vi "Analog Input Voltages.vi"(8 "error in (no error)":errorcluster, 10 "Analog Input Voltages":waveform(dbl)[](array[waveform]), 11 "BPG in":refnum<class "BPG.lvclass">) -> (0 "error out":errorcluster, 3 "BPG out":refnum<class "BPG.lvclass">)   [LabVIEW 2021, in "BPG.lvclass"]
uses:
  BPG.lvclass
  C:/Program Files/National Instruments/LabVIEW 2021/vi.lib/ActorFramework/Actor/Actor.lvclass
  <vilib>/NathanCo/Color Compare/Utilities/Colors.ctl
  BPG.lvclass/BPG.ctl
  <vilib>/ActorFramework/Actor/Actor.lvclass/Actor.ctl
  Pressure Gauges/Pressure Gauges Messages/Received Pressure Msg/Received Pressure Msg.lvclass/Received Pressure Msg.ctl
  <vilib>/ActorFramework/Message Enqueuer/Message Enqueuer.lvclass/Message Enqueuer.ctl
  <vilib>/ActorFramework/Message Enqueuer/Enqueue.vi
  Pressure Gauges/Pressure Gauges Messages/Received Pressure Msg/Received Pressure Msg.lvclass
  C:/Program Files/National Instruments/LabVIEW 2021/vi.lib/ActorFramework/Message/Message.lvclass
  <vilib>/ActorFramework/Message Priority Queue/Priority Enqueue.vi
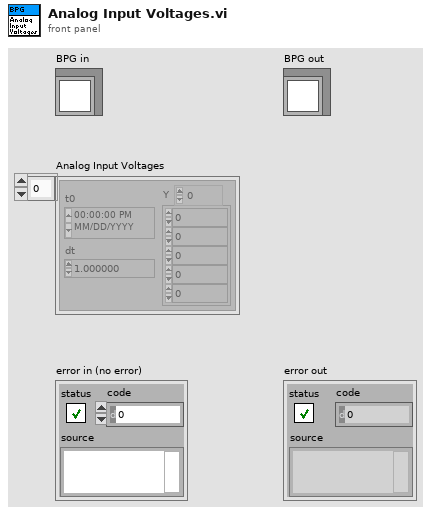
[diagram p1: front panel]
types:
  T1 = typedef "Colors.ctl" = cluster{"Green":u32, "Yellow":u32, "Red":u32}
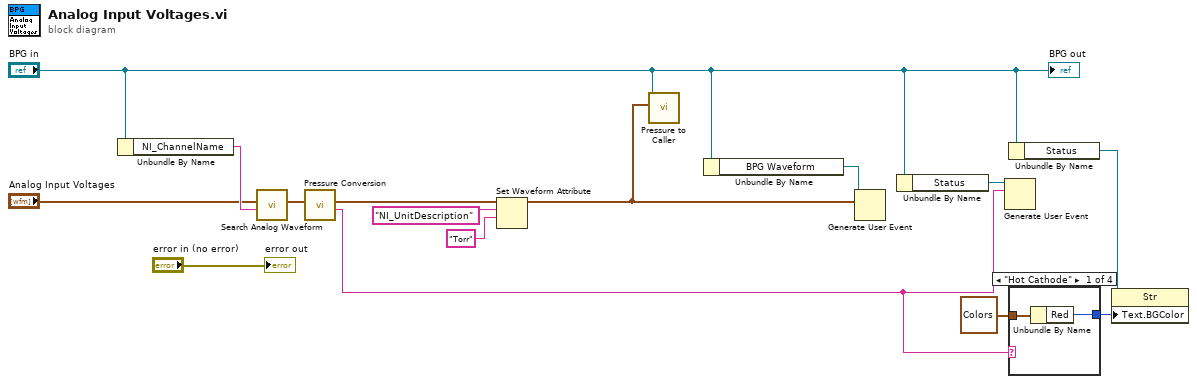
[diagram p0: block diagram]
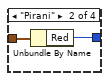
[diagram p2: hidden frame]
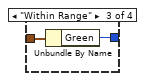
[diagram p3: hidden frame]
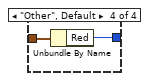
[diagram p4: hidden frame]
diagram:
  n1 = Unbundle By Name("BPG in") -> ("NI_ChannelName"=w8:string)
  n2 = call <vilib>:"Search Analog Waveform.vi"("NI_ChannelName"=w8, "Waveforms"="Analog Input Voltages") -> ("Waveform"=w7:waveform(dbl))  [unwired: 8 in, 1 out]
  n3 = call "Pressure Conversion.vi"("Waveform in"=w7) -> ("Status"=w5:string, "Waveform out"=w9:waveform(dbl))  [unwired: 9 in]
  n4 = Set Waveform Attribute(5:"Torr" ("name"), 6:"NI_UnitDescription" ("name"), 7:w9) -> (3:w1:waveform(dbl))  [unwired: 1 in, 2 out]
  n5 = call-dynamic "Pressure to Caller.vi"("Analog Input Waveform"=w1, "BPG in"="BPG in") -> ()  [unwired: 9 in, 1 out]
  n6 = Unbundle By Name("BPG in") -> ("BPG Waveform"=w15:refnum<user-event>)
  n7 = Generate User Event(user event=w15, event data cluster=w1) -> ()  [unwired: 2 in, 2 out]
  n8 = Unbundle By Name("BPG in") -> ("Status"=w14:refnum<user-event>)
  n9 = Generate User Event(user event=w14, event data cluster=w5) -> ()  [unwired: 2 in, 2 out]
  n10 = Unbundle By Name("BPG in") -> ("Status"=w13:refnum<vi>)
  n11 = case shown="\"Hot Cathode\"" w5 {
    tunnel: [w16 w18 w20 w23] -> w10
    tunnel: T1 {"Green"=65408, "Yellow"=16777088, "Red"=16744576} ("Colors") -> [w17 w19 w21 w22]
    frame "Hot Cathode" {
      n12 = Unbundle By Name(w17) -> ("Red"=w16:u32)
    }
    frame "Pirani" {
      n13 = Unbundle By Name(w19) -> ("Red"=w18:u32)
    }
    frame "Within Range" {
      n14 = Unbundle By Name(w21) -> ("Green"=w20:u32)
    }
    frame "Other", Default {
      n15 = Unbundle By Name(w22) -> ("Red"=w23:u32)
    }
  }
  n16 = property class="Str"(reference=w13, "Text.BGColor"=w10) -> ()  [unwired: 1 in, 2 out]
  "error out" <- "error in (no error)"
  "BPG out" <- "BPG in"
